vi "test_libssh2_session_flag.vi"() -> ()   [LabVIEW 2017, in "unit_tests.lvlib"]
uses:
  unit_tests.lvlib
  libssh2/libssh2_flag.ctl
  libssh2/libssh2_init_default.vi
  libssh2/libssh2_session_init_ex.vi
  libssh2/libssh2.lvlib
  <vilib>/PNR/Transparent Assertions/Transparent Assertions/Transparent Assertions.lvlib
panel:
  out "error out":errorcluster
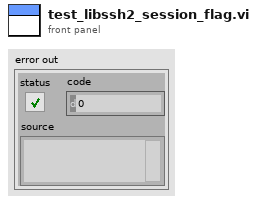
[diagram p1: front panel]
types:
  T1 = typedef "libssh2.lvlib/libssh2_flag.ctl" = enum16{"SIGPIPE", "COMPRESS", "QUOTE_PATHS"}
  T2 = typedef "libssh2.lvlib/Session Refnum.ctl" = refnum<k1>
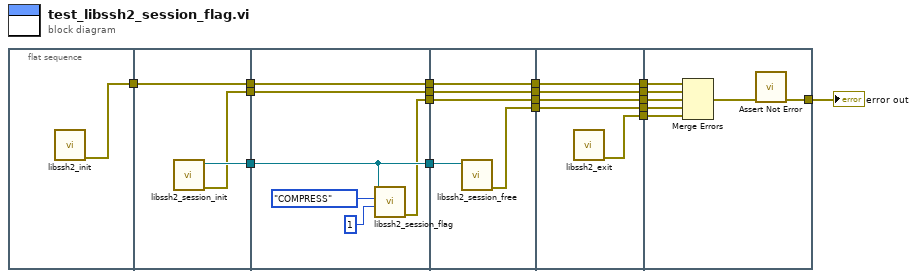
[diagram p0: block diagram]
diagram:
  n1 = flat-sequence {
    tunnel: [w19] -> w14
    tunnel: w14 -> [w22]
    tunnel: [w22] -> w9
    tunnel: [w21] -> w7
    tunnel: [w20] -> w5
    tunnel: w9 -> [w28]
    tunnel: [w28] -> w8
    tunnel: w7 -> [w25]
    tunnel: [w25] -> w6
    tunnel: w5 -> [w27]
    tunnel: [w27] -> w4
    tunnel: [w23] -> w3
    tunnel: w8 -> [w33]
    tunnel: [w33] -> w13
    tunnel: [w32] -> w12
    tunnel: w6 -> [w31]
    tunnel: w4 -> [w30]
    tunnel: [w30] -> w11
    tunnel: w3 -> [w29]
    tunnel: [w29] -> w2
    tunnel: w13 -> [w38]
    tunnel: [w38] -> w18
    tunnel: [w37] -> w17
    tunnel: [w36] -> w16
    tunnel: w12 -> [w36]
    tunnel: w11 -> [w35]
    tunnel: [w35] -> w10
    tunnel: w2 -> [w34]
    tunnel: [w34] -> w1
    tunnel: w18 -> [w45]
    tunnel: w17 -> [w44]
    tunnel: [w42] -> w15
    tunnel: w16 -> [w41]
    tunnel: w10 -> [w40]
    tunnel: w1 -> [w39]
    frame #0 {
      n2 = call-poly "libssh2_init.vi"() -> ("error out"=w19:errorcluster)  [unwired: 11 in]
    }
    frame #1 {
      n3 = call "libssh2_session_init.vi"() -> ("error out"=w20:errorcluster, "session"=w21:T2)  [unwired: 10 in]
    }
    frame #2 {
      n4 = call "libssh2_session_flag.vi"("value (0 = disabled)"=1, "flag"=libssh2_flag."COMPRESS", "session"=w25) -> ("error out"=w23:errorcluster)  [unwired: 8 in]
    }
    frame #3 {
      n5 = call "libssh2_session_free.vi"("session"=w31) -> ("error out"=w32:errorcluster)  [unwired: 10 in]
    }
    frame #4 {
      n6 = call "libssh2_exit.vi"() -> ("error out"=w37:errorcluster)  [unwired: 11 in]
    }
    frame #5 {
      n7 = Merge Errors(w45, w40, w39, w41, w44) -> (w43:errorcluster)
      n8 = call <vilib>:"Assert Not Error.vi"("error in (no error)"=w43) -> ("error out"=w42:errorcluster)  [unwired: 10 in]
    }
  }
  "error out" <- w15
